vi "ControlFotocelula_V1.vi"(0 "Tiempo de entrada a espera":timestamp) -> (1 "Aviso no detección":string, 2 "Boolean":bool)   [LabVIEW 2015]
panel:
  in  "Días sin detección de paso":dbl=3.0
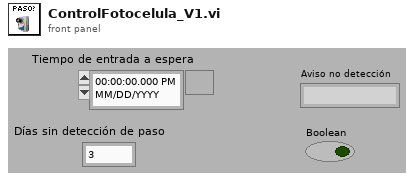
[diagram p1: front panel]
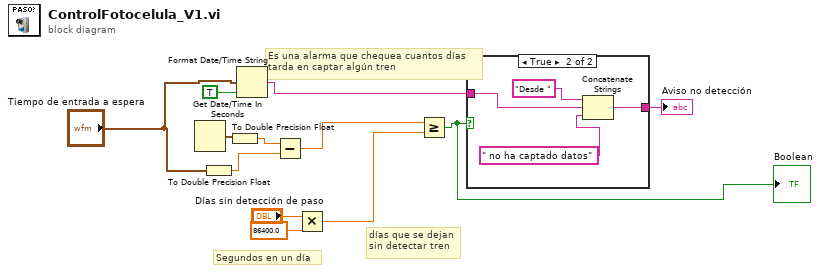
[diagram p0: block diagram]
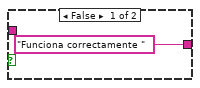
[diagram p2: hidden frame]
diagram:
  # "Segundos en un día"
  # "Es una alarma que chequea cuantos días\ntarda en captar algún tren"
  # "días que se dejan\nsin detectar tren"
  n1 = Get Date/Time In Seconds() -> (seconds since 1Jan1904=w7:timestamp)
  n2 = To Double Precision Float(number="Tiempo de entrada a espera") -> (double precision float=w3:dbl)
  n3 = To Double Precision Float(number=w7) -> (double precision float=w4:dbl)
  n4 = Format Date/Time String(seconds (now)="Tiempo de entrada a espera", UTC format=TRUE) -> (date/time string=w8:string)  [unwired: 1 in]
  n5 = Subtract(x=w4, y=w3) -> (x-y=w2:dbl)
  n6 = Multiply(x="Días sin detección de paso", y=86400.0) -> (x*y=w1:dbl)
  n7 = Greater Or Equal?(x=w2, y=w1) -> (x >= y?=w12:bool)
  "Boolean" <- w12
  n8 = case shown="True" w12 {
    tunnel: w8 -> [_ w16]
    tunnel: ["Funciona correctamente " ("String") w14] -> w11
    frame False {
    }
    frame True {
      n9 = Concatenate Strings("Desde " ("String"), w16, " no ha captado datos" ("String")) -> (w14:string)
    }
  }
  "Aviso no detección" <- w11
